vi "Control Intake.vi"(11 "loop time (ms)":u32) -> ()   [LabVIEW 2017]
uses:
  <vilib>/Rock Robotics/WPI/ThirdParty/Phoenix-LabVIEW/Motor Controller/Controls/CTRE_Phoenix_MotorControl_ControlMode.ctl
  <vilib>/Rock Robotics/WPI/Solenoid/WPI_SolenoidValue.ctl
  Globals/Robot Global Data.vi
  <vilib>/Rock Robotics/Network Tables/NT Write Boolean.vi
panel:
  in  "Dont Do Nick Thing Dont Want":bool
  in  "Intake Dont Hold Time":dbl=500.0
  in  "Cube Holding Voltage":dbl=0.175
  in  "Settle Time for Cube":dbl=0.5
  in  "Cube in Robot Threshold":dbl=2.5
  in  "Right Intake Scalar":dbl=1.0
  in  "Left Intake Scalar":dbl=1.0
  in  "Overall Intake Scalar":dbl=1.0
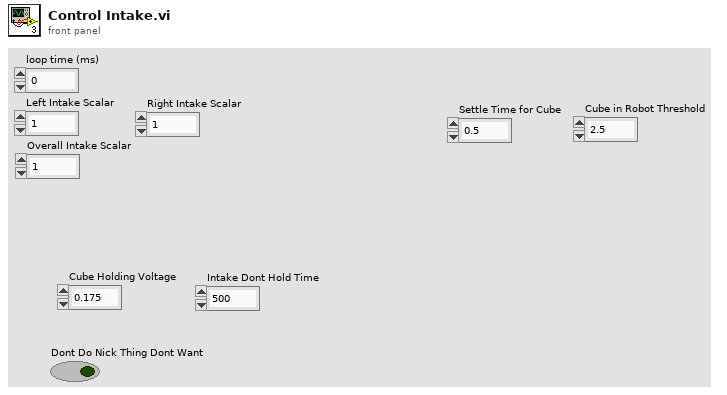
[diagram p1: front panel]
types:
  T1 = typedef "WPI_MotorControlDeviceRef.ctl" = cluster{"DeviceStatus":errorcluster, "Type":T2, "PWM":cluster{"PWM Channel":T3, "DeadBand":T4}, "CAN":cluster{"Device Number":u8, "SetOutput VI Ref":variant, "GetOutput VI Ref":variant, "Enable VI Ref":variant, "Disable VI Ref":variant, "Data":variant}, "Invert":bool, "DIO PWM":cluster{"PWM \"Enable\" Channel":T3, "DIOChannel":T5, "PWM Rate":dbl}}
  T2 = typedef "WPI_MotorControlType.ctl" = enum16{"PWM", "CAN", "DIO PWM"}
  T3 = typedef "FPGA_DIOPWMChannel.ctl" = enum8{"PWM 0", "PWM 1", "PWM 2", "PWM 3", "PWM 4", "PWM 5", "PWM 6", "PWM 7", "PWM 8", "PWM 9", "PWM MXP 0", "PWM MXP 1", "PWM MXP 2", "PWM MXP 3", "PWM MXP 4", "PWM MXP 5", "PWM MXP 6", "PWM MXP 7", "PWM MXP 8", "PWM MXP 9", "Invalid"}
  T4 = typedef "WPI_PWMDeadband.ctl" = cluster{"Name":string, "maxPositivePwm":i32, "minPositivePwm":i32, "centerPwm":i32, "maxNegativePwm":i32, "minNegativePwm":i32, "angularRange":u16}
  T5 = typedef "FPGA_DIOChannel.ctl" = enum8{"DIO 0", "DIO 1", "DIO 2", "DIO 3", "DIO 4", "DIO 5", "DIO 6", "DIO 7", "DIO 8", "DIO 9", "DIO MXP 0", "DIO MXP 1", "DIO MXP 2", "DIO MXP 3", "DIO MXP 4", "DIO MXP 5", "DIO MXP 6", "DIO MXP 7", "DIO MXP 8", "DIO MXP 9", "DIO MXP 10", "DIO MXP 11", "DIO MXP 12", "DIO MXP 13", "DIO MXP 14", "DIO MXP 15", "SPI Port CS1", "SPI Port CS2", "SPI Port CS3", "SPI Port MISO", "SPI Port MOSI", "Invalid"}
  T6 = typedef "WPI_SolenoidValue.ctl" = enum16{"Off", "On", "Forward", "Reverse"}
  T7 = typedef "CTRE_Phoenix_MotorControl_ControlMode.ctl" = u16
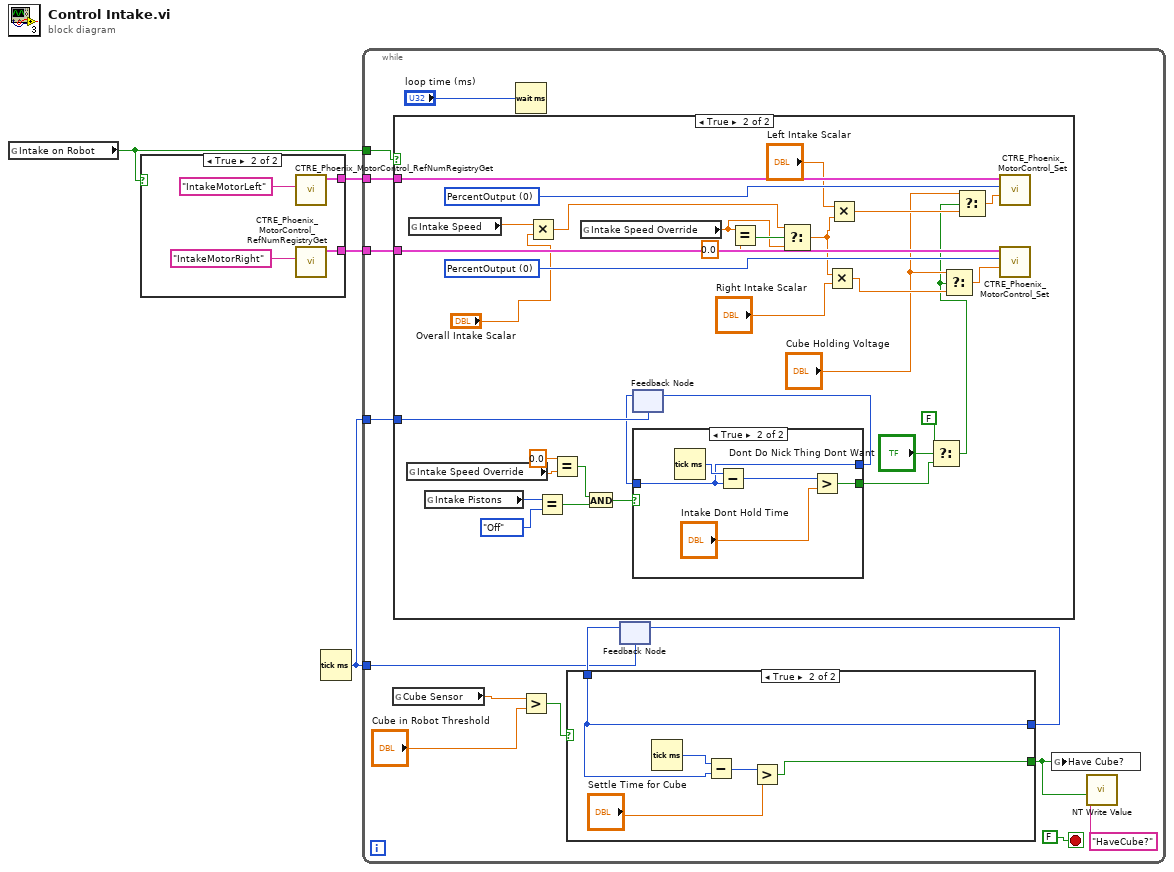
[diagram p0: block diagram]
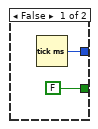
[diagram p3: hidden frame]
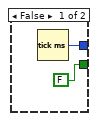
[diagram p5: hidden frame]
diagram:
  n1 = global read "Robot Global Data.vi" "Intake on Robot"() -> (w2:bool)
  n2 = case shown="True" w2 {
    tunnel: [_ w7] -> w4
    tunnel: [_ w6] -> w3
    frame False {
    }
    frame True {
      n3 = call "CTRE_Phoenix_MotorControl_RefNumRegistryGet.vi"("refnum name"="IntakeMotorLeft") -> ("PhoenixMotorControlDevRef"=w7:T1)  [unwired: 9 in, 1 out]
      n4 = call "CTRE_Phoenix_MotorControl_RefNumRegistryGet.vi"("refnum name"="IntakeMotorRight") -> ("PhoenixMotorControlDevRef"=w6:T1)  [unwired: 9 in, 1 out]
    }
  }
  n5 = Tick Count (ms)() -> (millisecond timer value=w1:u32)
  n6 = while {
    tunnel: w4 -> [w20]
    tunnel: w3 -> [w19]
    tunnel: w2 -> [w18]
    tunnel: w1 -> [w12]
    tunnel: w1 -> [w9]
    stop <- FALSE stop-if-true
    n7 = global read "Robot Global Data.vi" "Cube Sensor"() -> (w17:dbl)
    n8 = case shown="True" w18 {
      tunnel: w20 -> [_ w61]
      tunnel: w19 -> [_ w59]
      tunnel: w9 -> [_ w41]
      frame False {
      }
      frame True {
        w58 = T7 0 items=["PercentOutput"=0, "Position"=1, "Velocity"=2, "Current"=3, "Follower"=5, "MotionProfile"=6, "MotionMagic"=7, "MotionMagicArc"=8, "MotionProfileArc"=10, "Disabled"=15] ("Control Mode")
        w60 = T7 0 items=["PercentOutput"=0, "Position"=1, "Velocity"=2, "Current"=3, "Follower"=5, "MotionProfile"=6, "MotionMagic"=7, "MotionMagicArc"=8, "MotionProfileArc"=10, "Disabled"=15] ("Control Mode")
        n9 = global read "Robot Global Data.vi" "Intake Speed Override"() -> (w39:dbl)
        n10 = global read "Robot Global Data.vi" "Intake Speed"() -> (w57:dbl)
        n11 = global read "Robot Global Data.vi" "Intake Pistons"() -> (w38:T6)
        n12 = Multiply(x=w57, y="Overall Intake Scalar") -> (x*y=w53:dbl)
        n13 = Equal?(x=w38, y=WPI_SolenoidValue."Off" ("Intake Pistons")) -> (x = y?=w37:bool)
        n14 = Equal?(x=0.0, y=w39) -> (x = y?=w36:bool)
        n15 = global read "Robot Global Data.vi" "Intake Speed Override"() -> (w52:dbl)
        n16 = And(x=w36, y=w37) -> (x .and. y?=w35:bool)
        n17 = feedback #1(w41) -> (w40:u32)
        n18 = case shown="True" w35 {
          tunnel: w40 -> [_ w67]
          tunnel: [w63 w67] -> w42
          tunnel: [FALSE w65] -> w32
          frame False {
            n19 = Tick Count (ms)() -> (millisecond timer value=w63:u32)
          }
          frame True {
            n20 = Tick Count (ms)() -> (millisecond timer value=w68:u32)
            n21 = Subtract(x=w68, y=w67) -> (x-y=w66:u32)
            n22 = Greater?(x=w66, y="Intake Dont Hold Time") -> (0:w65:bool)
          }
        }
        n23 = feedback-in #1(w42) -> ()
        n24 = Equal?(x=w52, y=0.0) -> (x = y?=w54:bool)
        n25 = Select(t=w53, s=w54, f=w52) -> (s? t:f=w49:dbl)
        n26 = Multiply(x=w49, y="Right Intake Scalar") -> (x*y=w47:dbl)
        n27 = Multiply(x="Left Intake Scalar", y=w49) -> (x*y=w45:dbl)
        n28 = Select(t=FALSE, s="Dont Do Nick Thing Dont Want", f=w32) -> (s? t:f=w33:bool)
        n29 = Select(t="Cube Holding Voltage", s=w33, f=w47) -> (s? t:f=w48:dbl)
        n30 = Select(t="Cube Holding Voltage", s=w33, f=w45) -> (s? t:f=w46:dbl)
        n31 = call <vilib>:"CTRE_Phoenix_MotorControl_Set.vi"("Output"=w46, "Control Mode"=w60, "PhoenixMotorControlDevRef"=w61) -> ()  [unwired: 7 in, 2 out]
        n32 = call <vilib>:"CTRE_Phoenix_MotorControl_Set.vi"("Output"=w48, "Control Mode"=w58, "PhoenixMotorControlDevRef"=w59) -> ()  [unwired: 7 in, 2 out]
      }
    }
    n33 = Wait (ms)(milliseconds to wait="loop time (ms)") -> ()  [unwired: 1 out]
    n34 = Greater?(x=w17, y="Cube in Robot Threshold") -> (0:w15:bool)
    n35 = feedback #2(w12) -> (w13:u32)
    n36 = case shown="True" w15 {
      tunnel: w13 -> [_ w28]
      tunnel: [w24 w28] -> w14
      tunnel: [FALSE w26] -> w11
      frame False {
        n37 = Tick Count (ms)() -> (millisecond timer value=w24:u32)
      }
      frame True {
        n38 = Tick Count (ms)() -> (millisecond timer value=w29:u32)
        n39 = Subtract(x=w29, y=w28) -> (x-y=w27:u32)
        n40 = Greater?(x=w27, y="Settle Time for Cube") -> (0:w26:bool)
      }
    }
    n41 = feedback-in #2(w14) -> ()
    n42 = global write "Robot Global Data.vi" "Have Cube?"(w11) -> ()
    n43 = call-poly <vilib>:"NT Write Value.vi"("Boolean"=w11, "Name"="HaveCube?") -> ()  [unwired: 9 in, 1 out]
  }
